vi "Configure Multi Eval Meas Limit Emission Mask.vi"(0 "VISA resource name":refnum<visa-resource-name>, 1 "Enabled (Off)":bool, 2 "Frequency End (0Hz)":dbl format="%#.9p", 3 "RBW (\"M1\")":string="M1", 5 "Instance (1)":T3=1, 7 "Area (1)":T2=1, 9 "Bandwidth (5 MHz)":T1=5 items=["5 MHz"=5, "10 MHz"=10, "15 MHz"=15, "20 MHz"=20, "25 MHz"=25, "30 MHz"=30, "40 MHz"=40, "50 MHz"=50, "60 MHz"=60, "80 MHz"=80, "90 MHz"=90, "100 MHz"=100], 11 "error in (no error)":errorcluster, 12 "Frequency Start (0Hz)":dbl format="%#.9p", 13 "Level (0.0)":dbl format="%^.3e") -> (4 "VISA resource name out":refnum<visa-resource-name>, 15 "error out":errorcluster)   [LabVIEW 2020, in "Rohde&Schwarz CMWXP NR FR1 Measurement.lvlib"]
doc: "Defines general requirements for the emission mask area number <area> (for NR SA). The activation state, the area borders, an upper limit and the resolution bandwidth must be specified.\nThe emission mask applies to the channel bandwidth <bw>.\n\nAttribute:\nRSCMWXPNRFR1M_ATTR_MULTI_EVAL_MEAS_LIMIT_EMISSION_MASK\n\nRemote-control command:\nCONFigure:NRSub:MEAS<i>:MEValuation:LIMit:SEMask:AREA<area>:CBANdwidth<bw>"
uses:
  <instrlib>/Rohde&Schwarz CMWXP NR FR1 Measurement/Rohde&Schwarz CMWXP NR FR1 Measurement.lvlib
  <instrlib>/Rohde&Schwarz CMWXP NR FR1 Measurement/Private/_Instance.ctl
  <instrlib>/Rohde&Schwarz CMWXP NR FR1 Measurement/Private/_Area.ctl
  <instrlib>/Rohde&Schwarz CMWXP NR FR1 Measurement/Private/_Bandwidth.ctl
  <instrlib>/Rohde&Schwarz CMWXP NR FR1 Measurement/Private/rsidr_core.llb/rsidr_core.lvlib
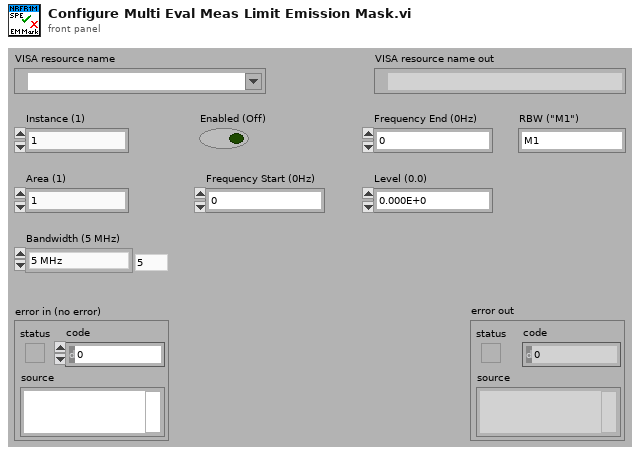
[diagram p1: front panel]
types:
  T1 = typedef "Rohde&Schwarz CMWXP NR FR1 Measurement.lvlib/_Bandwidth.ctl" = i32
  T2 = typedef "Rohde&Schwarz CMWXP NR FR1 Measurement.lvlib/_Area.ctl" = i32
  T3 = typedef "Rohde&Schwarz CMWXP NR FR1 Measurement.lvlib/_Instance.ctl" = i32
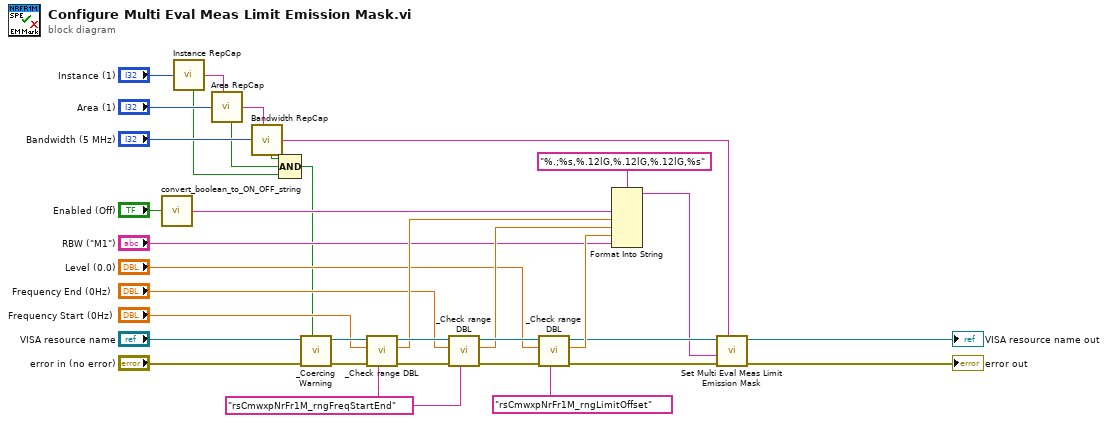
[diagram p0: block diagram]
diagram:
  w12 = "rsCmwxpNrFr1M_rngFreqStartEnd" ("Range Table Identifier")
  n1 = call <instrlib>:"convert_boolean_to_ON_OFF_string.vi"("boolean value in"="Enabled (Off)") -> ("string value out"=w26:string)  [unwired: 4 in]
  n2 = call <instrlib>:"Instance RepCap.vi"("Instance In"="Instance (1)") -> ("In Range?"=w4:bool, "RepCap Identifier Out"=w29:string)  [unwired: 1 in]
  n3 = call <instrlib>:"Area RepCap.vi"("SEM Area In"="Area (1)", "RepCap String In (\"\")"=w29) -> ("In Range?"=w3:bool, "RepCap Identifier Out"=w6:string)
  n4 = call <instrlib>:"Bandwidth RepCap.vi"("Bandwidth (5 MHz)"="Bandwidth (5 MHz)", "RepCap String In (\"\")"=w6) -> ("In Range?"=w2:bool, "RepCap Identifier Out"=w5:string)
  n5 = Compound Arithmetic op=AND(w2, w3, w4) -> (w1:bool)
  n6 = call <instrlib>:"_Coercing Warning.vi"("In Range?"=w1, "error in (no error)"="error in (no error)", "VISA resource name"="VISA resource name") -> ("error out"=w25:errorcluster, "VISA resource name out"=w24:refnum<visa-resource-name>)  [unwired: 7 in]
  n7 = call <instrlib>:"_Check range DBL.vi"("Range Table Identifier"=w12, "error in (no error)"=w25, "DBL Value In"="Frequency Start (0Hz)", "VISA resource name"=w24) -> ("error out"=w23:errorcluster, "DBL Value Out"=w18:dbl, "VISA resource name out"=w22:refnum<visa-resource-name>)  [unwired: 5 in]
  n8 = call <instrlib>:"_Check range DBL.vi"("Range Table Identifier"=w12, "error in (no error)"=w23, "DBL Value In"="Frequency End (0Hz)", "VISA resource name"=w22) -> ("error out"=w21:errorcluster, "DBL Value Out"=w16:dbl, "VISA resource name out"=w20:refnum<visa-resource-name>)  [unwired: 5 in]
  n9 = call <instrlib>:"_Check range DBL.vi"("Range Table Identifier"="rsCmwxpNrFr1M_rngLimitOffset", "error in (no error)"=w21, "DBL Value In"="Level (0.0)", "VISA resource name"=w20) -> ("error out"=w10:errorcluster, "DBL Value Out"=w14:dbl, "VISA resource name out"=w9:refnum<visa-resource-name>)  [unwired: 5 in]
  n10 = Format Into String(format string="%.;%s,%.12lG,%.12lG,%.12lG,%s", w26, w18, w16, w14, "RBW (\"M1\")") -> (resulting string=w8:string)  [unwired: 2 in, 1 out]
  n11 = call "Set Multi Eval Meas Limit Emission Mask"("Repeated Capabilities"=w5, "error in (no error)"=w10, "Multi Eval Meas Limit Emission Mask ()"=w8, "instrument handle"=w9) -> ("error out"=→"error out":errorcluster, "instrument handle out"=→"VISA resource name out":refnum<visa-resource-name>)  [unwired: 6 in]
